vi "nirviInterrupt.vi"(1 "Wait Until Cleared":bool, 2 "IRQ Number":u8) -> (0 "Error":bool)   [LabVIEW 2017]
doc: "Asserts an interrupt on the interrupt line of the FPGA target."
uses:
  <vilib>/rvi/interface/RandomDataEmulation/niFpgaIRQMethods.ctl
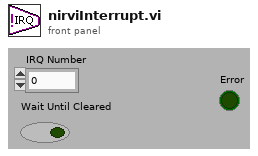
[diagram p1: front panel]
types:
  T1 = typedef "niFpgaIRQMethods.ctl" = enum16{"Get Array of IRQs", "Ack IRQ", "Assert IRQ"}
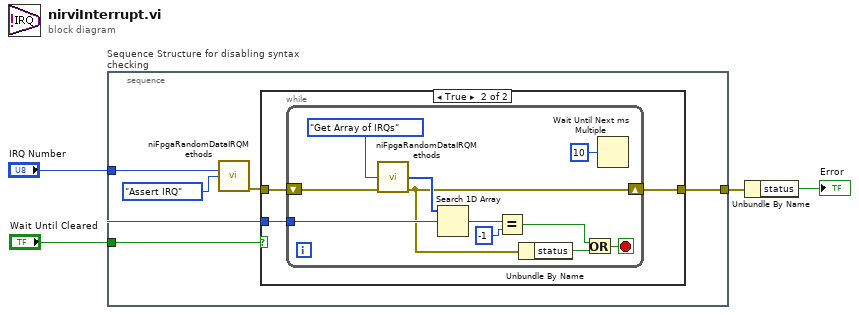
[diagram p0: block diagram]
diagram:
  n1 = stacked-sequence "Sequence Structure for disabling syntax checking" {
    tunnel: "IRQ Number" -> [w6]
    tunnel: "Wait Until Cleared" -> [w9]
    tunnel: [w8] -> w2
    frame #0 {
      n2 = call <vilib>:"niFpgaRandomDataIRQMethods.vi"("IRQ"=w6, "IRQ Method"=niFpgaIRQMethods."Assert IRQ") -> ("error out"=w7:errorcluster)  [unwired: 12 in, 1 out]
      n3 = case shown="True" w9 {
        tunnel: w7 -> [w10 w13]
        tunnel: [w10 w12] -> w8
        tunnel: w6 -> [_ w11]
        frame False {
        }
        frame True {
          n4 = while {
            shift-right: [w16] -> w12
            shift-left: w13 -> [w23]
            tunnel: w11 -> [w20]
            stop <- w24 stop-if-true
            n5 = call <vilib>:"niFpgaRandomDataIRQMethods.vi"("IRQ Method"=niFpgaIRQMethods."Get Array of IRQs", "error in (no error)"=w23) -> ("IRQ Array"=w21:u8[], "error out"=w16:errorcluster)  [unwired: 12 in]
            n6 = Search 1D Array(1D array=w21, element=w20) -> (index of element=w19:i32)  [unwired: 1 in]
            n7 = Equal?(x=w19, y=-1) -> (x = y?=w17:bool)
            n8 = Unbundle By Name(w16) -> ("status"=w22:bool)
            n9 = Or(x=w17, y=w22) -> (x .or. y?=w24:bool)
            n10 = Wait Until Next ms Multiple(millisecond multiple=u32 10) -> ()  [unwired: 1 out]
          }
        }
      }
    }
  }
  n11 = Unbundle By Name(w2) -> ("status"=→"Error":bool)
